vi "TECLADO_2009.vi"() -> ()   [LabVIEW 2019]
uses:
  CLASE SJD1/Variables Globales.vi
panel:
  in  "CORREGIR":bool
  out "incorrecto":string
  in  "1":bool
  in  "2":bool
  out "error out":errorcluster
  in  "error in (no error)":errorcluster
  in  "OK Button":bool
  in  "11":bool
  in  "9":bool
  in  "8":bool
  in  "7":bool
  in  "6":bool
  in  "5":bool caption="1 4"
  in  "4":bool
  in  "3":bool
  out "Result":string
  # "TECLADO"
  # "TÉCNICAS DE PROGRAMACIÓN"
  # "INTRODUZCA CÓDIGO"
  # "(C) 2009"
  # "CENTRO INTEGRADO DE FORMACIÓN PROFESIONAL número UNO"
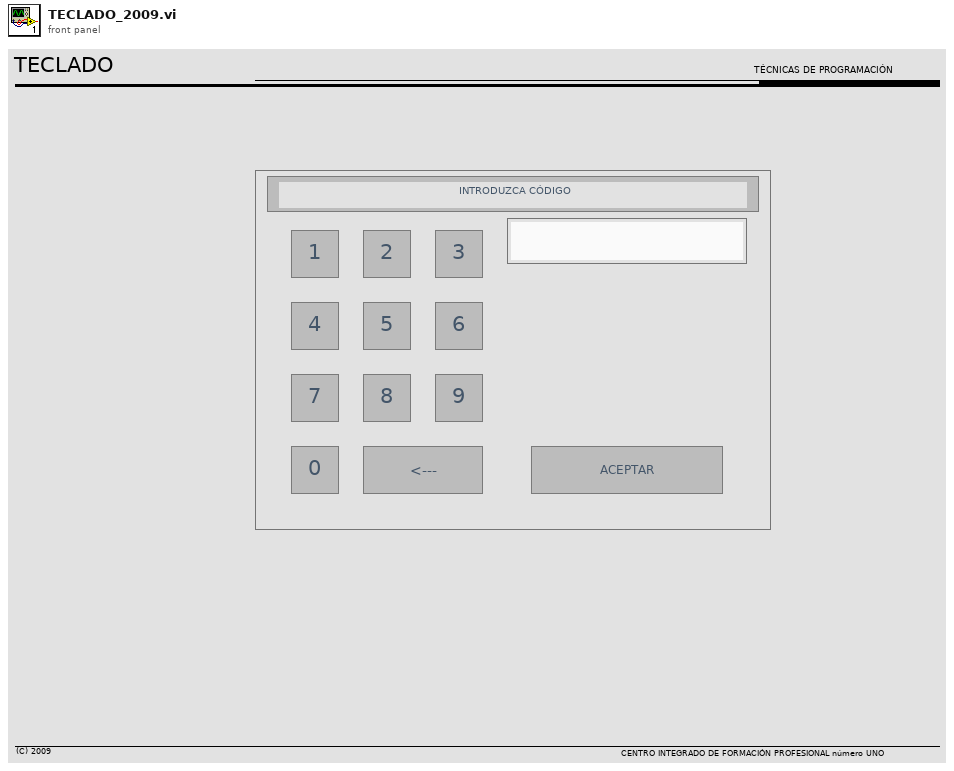
[diagram p1: front panel]
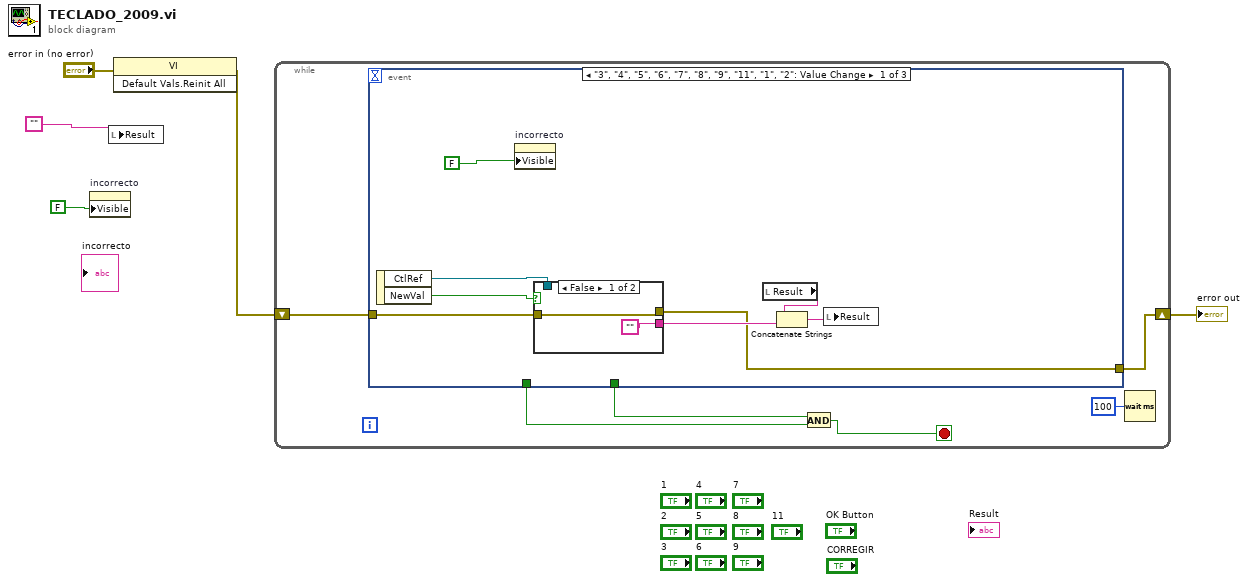
[diagram p0: block diagram]
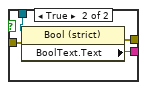
[diagram p2: hidden frame]
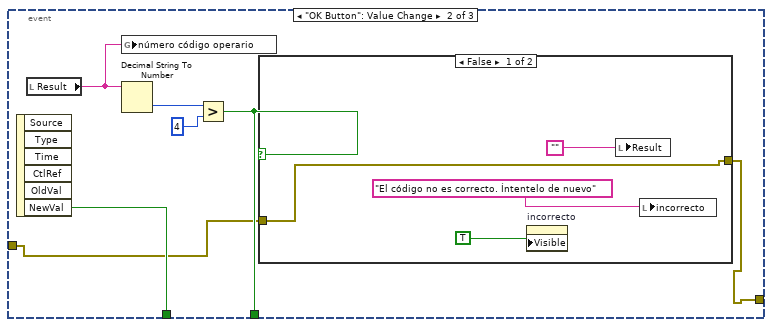
[diagram p3: hidden frame]
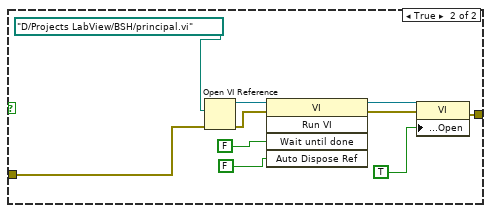
[diagram p4: hidden frame]
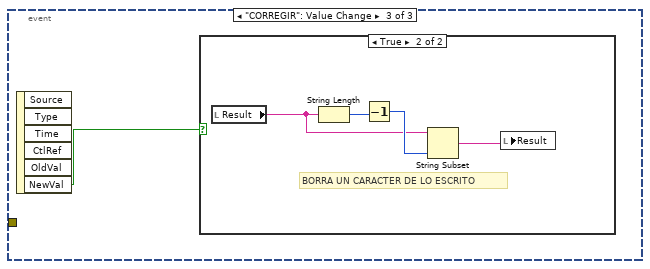
[diagram p5: hidden frame]
diagram:
  n1 = property on="incorrecto" class="Str"("Visible"=FALSE) -> ()  [unwired: 2 in, 2 out]
  n2 = local write "Result"("") -> ()
  n3 = invoke class="VI" method="Default Vals.Reinit All"(error in="error in (no error)") -> (error out=w1:errorcluster)  [unwired: 2 in, 2 out]
  n4 = while {
    shift-right: [w9] -> w3
    shift-left: w1 -> [w10]
    stop <- w8 stop-if-true
    n5 = event shown="[0] \"3\", \"4\", \"5\", \"6\", \"7\", \"8\", \"9\", \"11\", \"1\", \"2\": Value Change" {
      selector: _ -> [_ _ _]
      dyn-events: _ -> [_ _ _]
      timeout: _ -> [_ _ _]
      tunnel: w10 -> [w15 w28 _]
      tunnel: [w14 w27 _] -> w9
      tunnel: [_ w32 _] -> w7
      tunnel: [_ w29 _] -> w6
      event "3", "4", "5", "6", "7", "8", "9", "11", "1", "2": Value Change {
        n6 = event-data() -> ("CtlRef"=w19:refnum<vi>, "NewVal"=w13:bool)  [unwired: 1 out]
        n7 = property on="incorrecto" class="Str"("Visible"=FALSE) -> ()  [unwired: 2 in, 2 out]
        n8 = case shown="False" w13 {
          tunnel: w19 -> [_ w25]
          tunnel: ["" w24] -> w16
          tunnel: w15 -> [w21 w23]
          tunnel: [w21 w22] -> w14
          frame False {
          }
          frame True {
            n9 = property class="Bool (strict)"(reference=w25, error in=w23) -> (error out=w22:errorcluster, "BoolText.Text"=w24:string)  [unwired: 1 out]
          }
        }
        n10 = local read "Result"() -> (w17:string)
        n11 = Concatenate Strings(w17, w16) -> (w18:string)
        n12 = local write "Result"(w18) -> ()
      }
      event "OK Button": Value Change {
        n13 = event-data() -> ("NewVal"=w32:bool)  [unwired: 6 out]
        n14 = local read "Result"() -> (w26:string)
        n15 = global write "Variables Globales.vi" "número código operario"(w26) -> ()
        n16 = Decimal String To Number(string=w26) -> (number=w30:i32)  [unwired: 3 out]
        n17 = Greater?(x=w30, y=4) -> (0:w29:bool)
        n18 = case shown="False" w29 {
          tunnel: w28 -> [w34 w39]
          tunnel: [w34 w38] -> w27
          frame False {
            n19 = property on="incorrecto" class="Str"("Visible"=TRUE) -> ()  [unwired: 2 in, 2 out]
            n20 = local write "Result"("") -> ()
            n21 = local write "incorrecto"("El código no es correcto. Íntentelo de nuevo") -> ()
          }
          frame True {
            n22 = Open VI Reference(vi path=path "D:/Projects LabView/BSH/principal.vi", error in (no error)=w39) -> (vi reference=w41:refnum<vi>, error out=w40:errorcluster)  [unwired: 4 out]
            n23 = invoke class="VI" method="Run VI"(reference=w41, error in=w40, "Wait until done"=FALSE ("Wait Until Done"), "Auto Dispose Ref"=FALSE ("Auto Dispose Reference")) -> (reference out=w44:refnum<vi>, error out=w45:errorcluster)  [unwired: 1 in, 3 out]
            n24 = property class="VI"(reference=w44, error in=w45, "Front Panel.Open"=TRUE ("Front Panel Window:Open")) -> (error out=w38:errorcluster)  [unwired: 1 out]
          }
        }
      }
      event "CORREGIR": Value Change {
        n25 = event-data() -> ("NewVal"=w47:bool)  [unwired: 6 out]
        n26 = case shown="True" w47 {
          frame False {
          }
          frame True {
            # "BORRA UN CARACTER DE LO ESCRITO"
            n27 = local read "Result"() -> (w49:string)
            n28 = String Length(string=w49) -> (length=w50:i32)
            n29 = Decrement(x=w50) -> (x-1=w51:i32)
            n30 = String Subset(string=w49, length (rest)=w51) -> (substring=w48:string)  [unwired: 1 out]
            n31 = local write "Result"(w48) -> ()
          }
        }
      }
    }
    n32 = And(x=w6, y=w7) -> (x .and. y?=w8:bool)
    n33 = Wait (ms)(milliseconds to wait=u32 100) -> ()  [unwired: 1 out]
  }
  "error out" <- w3
